vi "Content.vi"(7 "Context":refnum<class "Context.lvclass">, 8 "Error In":errorcluster, 11 "Text In":refnum<class "Text.lvclass">) -> (0 "Error Out":errorcluster, 2 "Content":string, 3 "Text Out":refnum<class "Text.lvclass">)   [LabVIEW 2018, in "Toolkit.lvlib" / "Nodes.lvlib" / "Text.lvclass"]
uses:
  Text.lvclass
  Support/Context/Context.lvclass
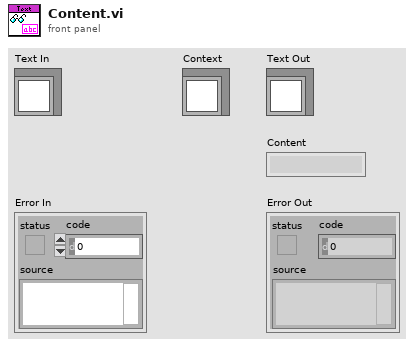
[diagram p1: front panel]
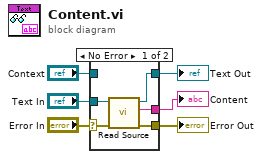
[diagram p0: block diagram]
diagram:
  n1 = case shown="No Error" "Error In" {
    selector: "Error In" -> [w8 w13]
    tunnel: [w9 w13] -> w5
    tunnel: "Text In" -> [w11 w12]
    tunnel: [w10 w12] -> w3
    tunnel: "Context" -> [_ _]
    tunnel: [w7 _] -> w1
    frame No Error {
      n2 = call-dynamic "Read Source.vi"("Error In"=w8, "Node In"=w11) -> ("Error Out"=w9:errorcluster, "Source"=w7:string, "Node Out"=w10:refnum<class "Text.lvclass">)  [unwired: 7 in]
    }
    frame Error {
    }
  }
  "Error Out" <- w5
  "Text Out" <- w3
  "Content" <- w1
